vi "Wf ascii to float.vi"(10 "String array":string) -> (2 "Array out":dbl[](array[numeric]))   [LabVIEW 2010, in "RedPitaya.lvlib"]
doc: "Takes ASCII format read data from Red Pitaya buffer and converts it into double value array."
uses:
  RedPitaya.lvlib
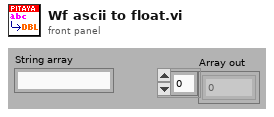
[diagram p1: front panel]
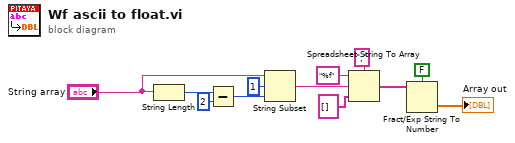
[diagram p0: block diagram]
diagram:
  n1 = String Length(string="String array") -> (length=w5:i32)
  n2 = Subtract(x=w5, y=2) -> (x-y=w6:i32)
  n3 = String Subset(string="String array", offset (0)=1, length (rest)=w6) -> (substring=w3:string)
  n4 = Spreadsheet String To Array(delimiter (Tab)=",", format string="%f", spreadsheet string=w3, array type (2D Dbl)=string[] [] ("Array")) -> (array=w9:string[])
  n5 = Fract/Exp String To Number(use system decimal point (T)=FALSE, string=w9) -> (number=→"Array out":dbl[])  [unwired: 3 out]
